vi "Input Register Get Data Type.vi"(8 "error in (no error)":errorcluster, 11 "Item Ref in":T2 format="%.0x") -> (0 "error out":errorcluster, 2 "Data Type":T1, 3 "Item Ref out":T2 format="%.0x")   [LabVIEW 2015, in "Modbus Master System Explorer.lvlib"]
uses:
  Modbus Master System Explorer.lvlib
  <vilib>/NI Veristand/Custom Device API/Custom Device Item Ref.ctl
  Shared/Controls/Data Model/DataType.ctl
  Shared/Constants.vi
  <vilib>/NI Veristand/Custom Device API/Get Item Property (U16).vi
  <vilib>/NI VeriStand/Custom Device API/Custom Device API.lvlib
  Shared/Modbus Master Shared.lvlib
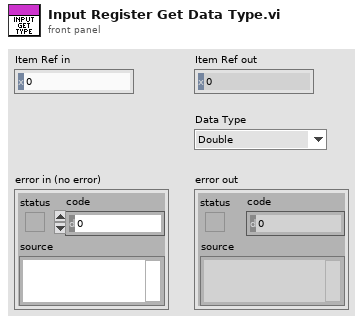
[diagram p1: front panel]
types:
  T1 = typedef "Modbus Master Shared.lvlib/DataType.ctl" = enum16{"Double", "Single", "I64", "I32", "I16", "I8", "U64", "U32", "U16", "U8", "Boolean"}
  T2 = typedef "Custom Device API.lvlib/Custom Device Item Ref.ctl" = u64
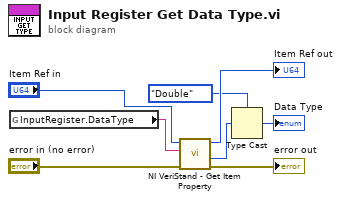
[diagram p0: block diagram]
diagram:
  n1 = global read "Constants.vi" "InputRegister.DataType"() -> (w8:string)
  n2 = call-poly <vilib>:"NI VeriStand - Get Item Property.vi"("error in (no error)"="error in (no error)", "Property Name"=w8, "Item Ref in"="Item Ref in") -> ("error out"=→"error out":errorcluster, "Value"=w2:u16, "Item Ref out"=→"Item Ref out":T2)  [unwired: 5 in, 1 out]
  n3 = Type Cast(type=DataType."Double" ("DataType"), x=w2) -> (*(type *) &x=→"Data Type":T1)
